vi "Launch Subordinate and Add.vi"(8 "error in":errorcluster, 9 "Panel Definiton":T1, 10 "Identifier":string, 11 "Manual UI in":refnum<class "Manual UI.lvclass">) -> (0 "error out":errorcluster, 3 "Manual UI out":refnum<class "Manual UI.lvclass">)   [LabVIEW 2019, in "Manual UI.lvlib" / "Manual UI.lvclass"]
uses:
  Project/Manual UI.lvclass
  builds/Engine/Panel Manager.lvlibp/Panel Actor/Panel Actor.lvclass
  builds/Engine/Panel.lvlibp/Panel/Panel.lvclass
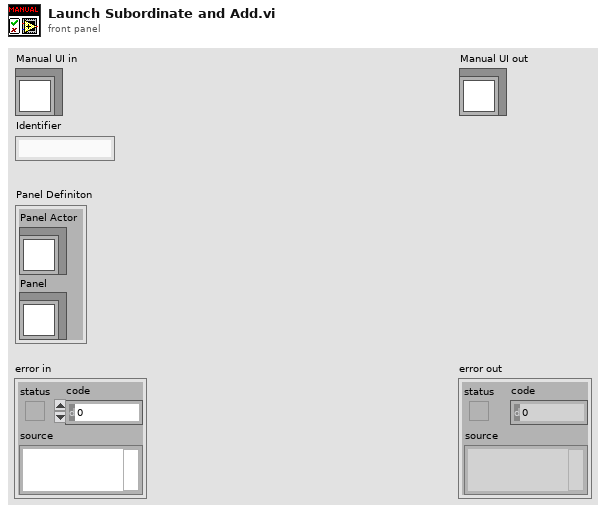
[diagram p1: front panel]
types:
  T1 = cluster{"Panel Actor":refnum<class "Panel Actor.lvclass">, "Panel":refnum<class "Panel.lvclass">}
  T2 = cluster{"Identifier":string, "Enqueuer":refnum<class "Message Enqueuer.lvclass">}
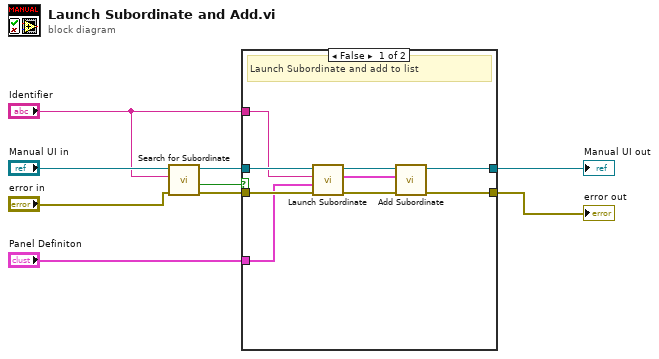
[diagram p0: block diagram]
diagram:
  n1 = call "Search for Subordinate.vi"("error in"="error in", "Identifier"="Identifier", "Manual UI in"="Manual UI in") -> ("error out"=w4:errorcluster, "Found"=w7:bool, "Manual UI out"=w6:refnum<class "Manual UI.lvclass">)  [unwired: 4 in, 2 out]
  n2 = case shown="False" w7 {
    tunnel: w6 -> [w17 w20]
    tunnel: [w11 w20] -> w5
    tunnel: w4 -> [w18 w19]
    tunnel: [w10 w19] -> w3
    tunnel: "Identifier" -> [w16 _]
    tunnel: "Panel Definiton" -> [w15 _]
    frame False {
      # "Launch Subordinate and add to list"
      n3 = call "Launch Subordinate.vi"("error in"=w18, "Panel Definiton"=w15, "Identifier"=w16, "Manual UI in"=w17) -> ("error out"=w14:errorcluster, "Subordinate"=w12:T2, "Manual UI out"=w13:refnum<class "Manual UI.lvclass">)  [unwired: 5 in]
      n4 = call "Add Subordinate.vi"("error in"=w14, "Subordinate"=w12, "Manual UI in"=w13) -> ("error out"=w10:errorcluster, "Manual UI out"=w11:refnum<class "Manual UI.lvclass">)  [unwired: 7 in]
    }
    frame True {
      # "Actor Found, Do nothing"
    }
  }
  "error out" <- w3
  "Manual UI out" <- w5
